vi "SimplifiedCounter_2.vi"() -> ()   [LabVIEW 2020]
uses:
  <vilib>/Platform/TimedLoop/XDataNode/timing_clust.ctl
  <vilib>/Platform/TimedLoop/XDataNode/nitl_modes.ctl
  <vilib>/Platform/TimedLoop/XDataNode/wakeup.ctl
  <vilib>/rvi/Emulation/niFpgaGetClockAttributes.vi
  <vilib>/rvi/Emulation/niFpgaSctlEmulationGetInTimedLoop.vi
  <vilib>/rvi/Emulation/niFpgaEmulationReportErrorSimple.vi
  <vilib>/rvi/DataTransferAndStorage/Container/Common/niFpgaContainerExecOnDevCompGetState.vi
  <vilib>/rvi/Emulation/niFpgaEmulationIsFPGAContextNoSignature.vi
  <vilib>/rvi/errors/niFpgaSetErrorForExecOnDevCompSimple.vi
  <vilib>/rvi/eio/common/nirviEmuReportErrorAndStop.vi
  <vilib>/rvi/DataTransferAndStorage/Container/Common/niFpgaContainerGetUniqueNameForEmu.vi
  <vilib>/rvi/FIFO/Fifo_Resource/nirvififoEmulationSetSize.vi
  <vilib>/rvi/FIFO/Fifo_Resource/nirviFifoEmulationQueueMgr.vi
  <instcachedir>/0/nirviFifoEmulationQueueMgr_E5CAEC123FF24DC58D834DCA3CDAA9B5.lvgen/nirviFifoEmulationQueueMgr_E5CAEC123FF24DC58D834DCA3CDAA9B5_001.vi
  <vilib>/rvi/FIFO/Fifo_Resource/nirvififoEmulationDetermineInputValidOut.vi
  <vilib>/rvi/FIFO/Fifo_Resource/nirvififoEmulationCreateLock.vi
  <vilib>/rvi/Emulation/niFpgaProcessEmulError.vi
  <vilib>/rvi/FIFO/Fifo_Resource/nirvififoEmulationObtainLock.vi
  <vilib>/rvi/FIFO/Fifo_Resource/nirvififoEmulationReleaseLock.vi
  <vilib>/rvi/occurrence/nirviWaitOnOccurrenceBase.vi
  <vilib>/rvi/errors/nirviReportUnexpectedCaseInternalError.vi
  <vilib>/rvi/errors/nirviReportUnexpectedCaseInternalError (U32).vi
  <vilib>/Utility/error.llb/Clear Errors.vi
  <vilib>/rvi/interface/RandomDataEmulation/niFpgaRandomDataHandleErrors.vi
  <vilib>/rvi/Emulation/niFpgaCriticalErrorInLSC.vi
  <vilib>/rvi/eio/common/nirviEmuTemplateMethod_errors.vi
  <vilib>/rvi/DataTransferAndStorage/Container/XNode/niFpgaContainer.xnode
  <vilib>/rvi/FIFO/Fifo_Resource/niFpgaFifoEmulationRefIn.vi
  <vilib>/Platform/TimedLoop/XDataNode/XDataNode.xnode
  <vilib>/eio/EIONode/EIONode.xnode
  <vilib>/Platform/TimedLoop/XDataNode/XDNodeRunTimeDep.lvlib
panel:
  out "FIFO in":i16
  in  "FIFO In":refnum<k21>="FIFO_host2target"
  in  "Count(Ticks)":u32
  out "Counts":u32
  in  "Reset Counter":bool
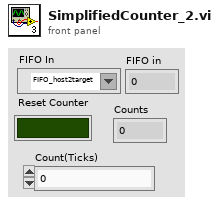
[diagram p1: front panel]
types:
  T1 = enum16{"Rising Edge", "Falling Edge", "Rising AND Falling Edges"}
  T2 = typedef "XDNodeRunTimeDep.lvlib/timing_clust.ctl" = cluster{"Expected End [f-1]":u64, "Actual End [f-1]":u64, "Finished Late? [f-1]":bool, "Expected End [i-1]":u64, "Actual End [i-1]":u64, "Finished Late? [i-1]":bool, "Expected Start [i]":u64, "Actual Start [i]":u64, "Expected Start [f]":u64, "Actual Start [f]":u64, "Source Name":string, "Structure Name":string, "Period":i64, "Deadline":i64, "Offset":i64, "Start":i64, "Priority":i32, "Timeout":i32, "Mode":T3, "Wakeup Reason":T4, "Error":errorcluster, "Source Type":string, "Secondary Source Type":string, "Global End Time":u64, "Global Start Time":u64, "Frame Duration":u64, "Iteration Duration":u64, "Assigned CPU":i32, "I/O Scan Engine Mode":u32}
  T3 = typedef "XDNodeRunTimeDep.lvlib/nitl_modes.ctl" = enum32{"No Change", "Process missed periods, maintain original phase", "Discard missed periods, maintain original phase", "Process missed periods, ignore original phase", "Discard missed periods, ignore original phase"}
  T4 = typedef "XDNodeRunTimeDep.lvlib/wakeup.ctl" = enum32{"Normal", "Aborted", "Asynchronous wakeup", "Timing source error", "Timed loop error", "Timeout"}
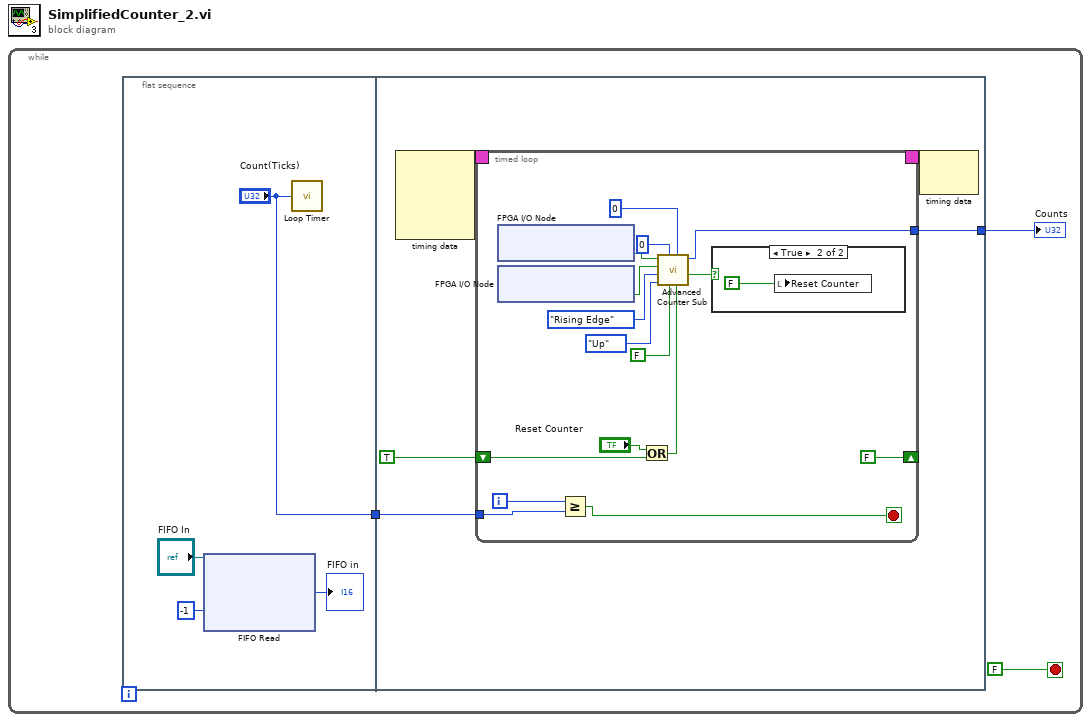
[diagram p0: block diagram]
diagram:
  n1 = while {
    stop <- FALSE stop-if-true
    n2 = flat-sequence {
      tunnel: ["Count(Ticks)"] -> w3
      tunnel: w3 -> [w12]
      tunnel: [w8] -> w1
      frame #0 {
        n3 = xnode "FIFO Read"("Timeout"=-1, "FIFO In"="FIFO In") -> ("Element"=→"FIFO in":i16)  [unwired: 2 out]
        n4 = call "Loop Timer"("Count(Ticks)"="Count(Ticks)") -> ()  [unwired: 1 out]
      }
      frame #1 {
        n5 = node-c288() -> (w11:T2)  [unwired: 4 in]
        n6 = timed-loop {
          timing: w11 -> [_]
          timing-out: [_] -> w10
          shift-right: [FALSE] -> _
          shift-left: TRUE -> [w21]
          tunnel: w12 -> [w15]
          tunnel: [w13] -> w8
          i -> [w16]
          stop <- w14 stop-if-true
          n7 = xnode "FPGA I/O Node"() -> ("Connector0/DIO0"=w28:bool)  [unwired: 1 in, 1 out]
          n8 = xnode "FPGA I/O Node"() -> ("Connector0/DIO1"=w27:bool)  [unwired: 1 in, 1 out]
          n9 = Greater Or Equal?(x=w16, y=w15) -> (x >= y?=w14:bool)
          n10 = Or(x="Reset Counter", y=w21) -> (x .or. y?=w17:bool)
          n11 = call "Advanced Counter Sub.vi"("Reset Counter"=w17, "Init Counter Value"=u32 0 ("Counter 0:Initial Count"), "Enable HW Gate"=FALSE ("Counter 0:Enable HW Gate"), "Ticks to Filter"=u32 0 ("Counter 0:Ticks to Filter"), "Count Direction"=enum16{"Up", "Down"}."Up" ("Counter 0:Count Direction"), "Edge"=T1."Rising Edge" ("Counter 0:Edge"), "Gate Signal"=w27, "Input Signal"=w28) -> ("Counter Reset?"=w18:bool, "Counter Out"=w13:u32)  [unwired: 2 in]
          n12 = case shown="True" w18 {
            frame False {
            }
            frame True {
              n13 = local write "Reset Counter"(FALSE ("Reset Counter")) -> ()
            }
          }
        }
        n14 = node-c288(w10) -> ()  [unwired: 1 out]
      }
    }
    "Counts" <- w1
  }
